vi "Begin.vi"(8 "error in":errorcluster) -> (0 "error out":errorcluster)   [LabVIEW 2020]
doc: "Called before other user functions, this VI is expected to open initial I/O refnums, load in file data, and do all program initialization. Notice that the <B>error out</B> terminal is simply used for data flow. Wiring it to other structures or subVIs ensures that this VI runs first."
uses:
  <vilib>/Rock Robotics/WPI/DriverStation/WPI_DriverStationRobotMode2.ctl
  <vilib>/Rock Robotics/WPI/Joystick/WPI_JoystickDeviceEnum.ctl
  <vilib>/Rock Robotics/WPI/RobotDrive/WPI_RobotDriveDevRef.ctl
  <vilib>/Rock Robotics/WPI/MotorControl/WPI_MotorControlDeviceRef.ctl
  <vilib>/Rock Robotics/WPI/MotorControl/WPI_MotorControlType.ctl
  <vilib>/Rock Robotics/SystemInterfaces/DIO/FPGA_DIOPWMChannel.ctl
  <vilib>/Rock Robotics/WPI/PWM/WPI_PWMDeadband.ctl
  <vilib>/Rock Robotics/SystemInterfaces/DIO/FPGA_DIOChannel.ctl
  <vilib>/Rock Robotics/WPI/SafetyOutput/WPI_SafetyOutputConfigMenu.ctl
  <vilib>/Rock Robotics/WPI/Solenoid/WPI_SolenoidChannel.ctl
  <vilib>/Rock Robotics/WPI/ThirdParty/REV Robotics/REVLib/Typedef/Spark MAX Idle Mode.ctl
  <vilib>/Rock Robotics/WPI/ThirdParty/REV Robotics/REVLib/Typedef/Spark MAX Motor Type.ctl
  Robot Global Data.vi
  <vilib>/Rock Robotics/Network Tables/NT Write String Array.vi
  <vilib>/Rock Robotics/WPI/Utilities/WPI_GetSetVariantRefNum.vi
  <vilib>/Rock Robotics/WPI/Solenoid/WPI_SolenoidOpenSingle.vi
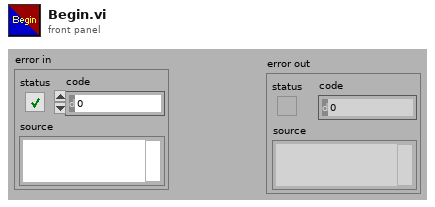
[diagram p1: front panel]
types:
  T1 = typedef "WPI_SafetyOutputConfigMenu.ctl" = enum16{"Enable", "Disable"}
  T2 = typedef "WPI_SolenoidChannel.ctl" = enum8{"Solenoid 0", "Solenoid 1", "Solenoid 2", "Solenoid 3", "Solenoid 4", "Solenoid 5", "Solenoid 6", "Solenoid 7", "Solenoid 8", "Solenoid 9", "Solenoid 10", "Solenoid 11", "Solenoid 12", "Solenoid 13", "Solenoid 14", "Solenoid 15", "Invalid"}
  T3 = typedef "WPI_JoystickDeviceEnum.ctl" = enum16{"USB 0", "USB 1", "USB 2", "USB 3", "USB 4", "USB 5"}
  T4 = typedef "WPI_RobotDriveDevRef.ctl" = cluster{"DevStatus":errorcluster, "Motors[]":T5[], "Square Inputs":bool, "Max Output":dbl}
  T5 = typedef "WPI_MotorControlDeviceRef.ctl" = cluster{"DeviceStatus":errorcluster, "Type":T6, "PWM":cluster{"PWM Channel":T7, "DeadBand":T8}, "CAN":cluster{"Device Number":u8, "SetOutput VI Ref":variant, "GetOutput VI Ref":variant, "Enable VI Ref":variant, "Disable VI Ref":variant, "Data":variant}, "Invert":bool, "DIO PWM":cluster{"PWM \"Enable\" Channel":T7, "DIOChannel":T9, "PWM Rate":dbl}}
  T6 = typedef "WPI_MotorControlType.ctl" = enum16{"PWM", "CAN", "DIO PWM"}
  T7 = typedef "FPGA_DIOPWMChannel.ctl" = enum8{"PWM 0", "PWM 1", "PWM 2", "PWM 3", "PWM 4", "PWM 5", "PWM 6", "PWM 7", "PWM 8", "PWM 9", "PWM MXP 0", "PWM MXP 1", "PWM MXP 2", "PWM MXP 3", "PWM MXP 4", "PWM MXP 5", "PWM MXP 6", "PWM MXP 7", "PWM MXP 8", "PWM MXP 9", "Invalid"}
  T8 = typedef "WPI_PWMDeadband.ctl" = cluster{"Name":string, "maxPositivePwm":i32, "minPositivePwm":i32, "centerPwm":i32, "maxNegativePwm":i32, "minNegativePwm":i32, "angularRange":u16}
  T9 = typedef "FPGA_DIOChannel.ctl" = enum8{"DIO 0", "DIO 1", "DIO 2", "DIO 3", "DIO 4", "DIO 5", "DIO 6", "DIO 7", "DIO 8", "DIO 9", "DIO MXP 0", "DIO MXP 1", "DIO MXP 2", "DIO MXP 3", "DIO MXP 4", "DIO MXP 5", "DIO MXP 6", "DIO MXP 7", "DIO MXP 8", "DIO MXP 9", "DIO MXP 10", "DIO MXP 11", "DIO MXP 12", "DIO MXP 13", "DIO MXP 14", "DIO MXP 15", "SPI Port CS1", "SPI Port CS2", "SPI Port CS3", "SPI Port MISO", "SPI Port MOSI", "Invalid"}
  T10 = typedef "WPI_DriverStationRobotMode2.ctl" = enum16{"Autonomous Disabled", "Autonomous Enabled", "Teleop Disabled", "Teleop Enabled", "Disconnected", "Finish", "Test Disabled", "Test Enabled", "Emergency Stopped"}
  T11 = typedef "WPI_SolenoidDevRef.ctl" = cluster{"DevStatus":errorcluster, "Pneumatics Control Module":u8, "Forward Solenoid Channel":T2, "Reverse Solenoid Channel":T2}
  T12 = typedef "WPI_CompressorDevRef.ctl" = cluster{"DevStatus":errorcluster, "Pneumatics Control Module":u8}
  T13 = typedef "WPI_JoystickDevRef.ctl" = cluster{"Device":T3}
  T14 = typedef "Spark MAX Motor Type.ctl" = enum16{"Brushed", "Brushless"}
  T15 = typedef "Spark MAX Idle Mode.ctl" = enum16{"Coast", "Brake"}
  T16 = cluster{"Motors[][0]":T5, "Motors[][1]":T5, "Motors[][2]":T5, "Motors[][3]":T5, "Motors[][4]":T5, "Motors[][5]":T5, "Motors[][6]":T5, "Motors[][7]":T5, "Motors[][8]":T5}
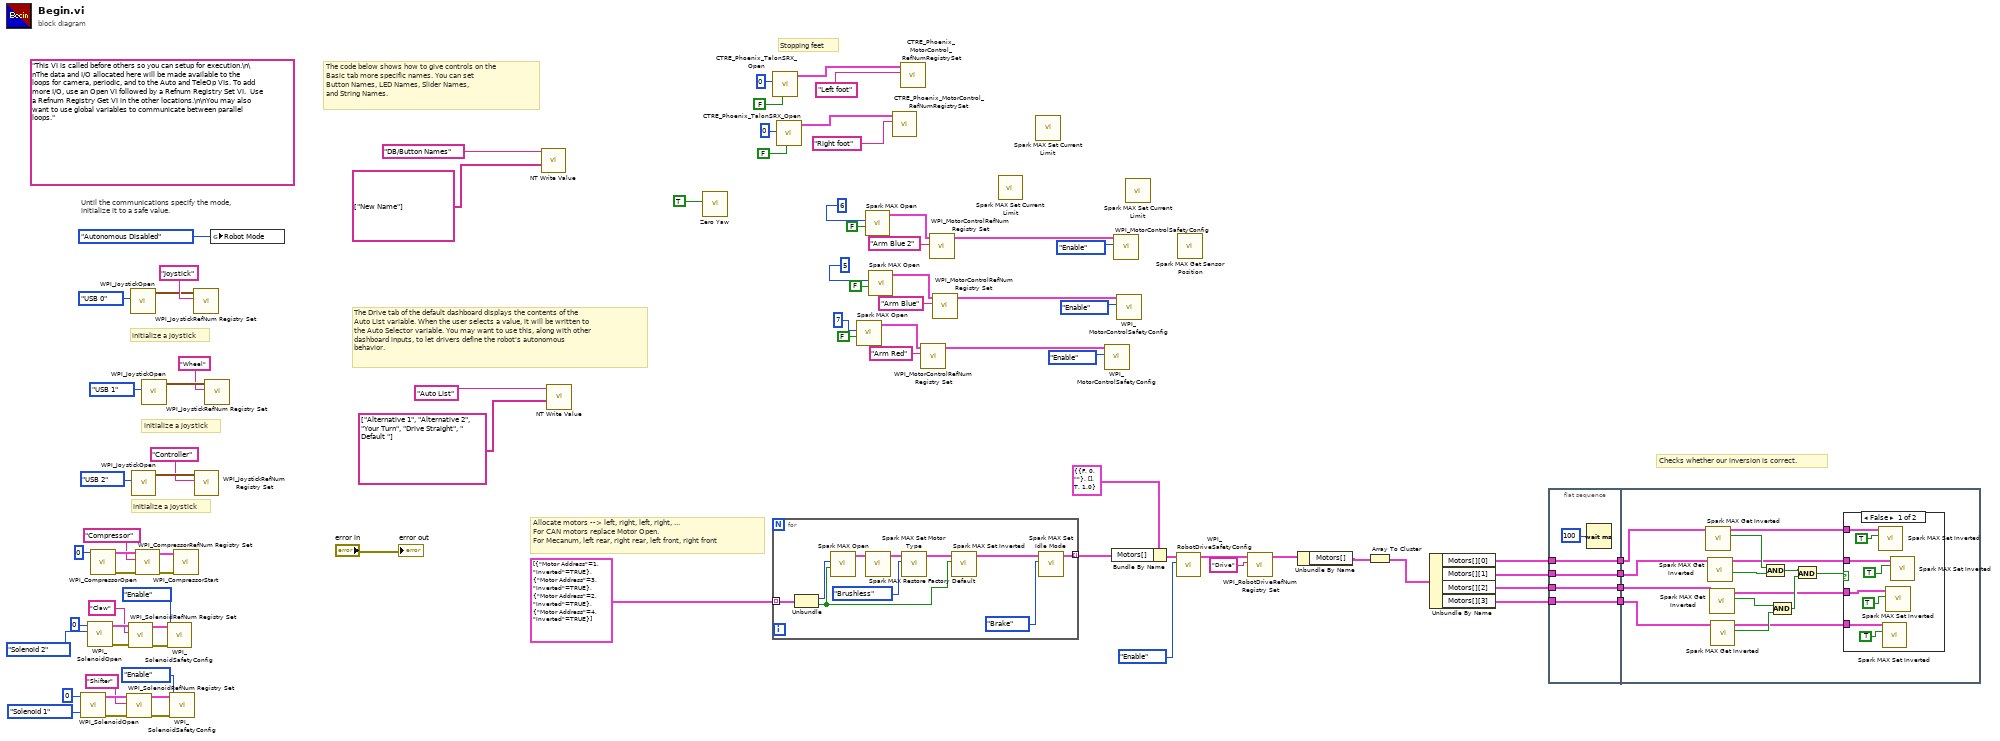
[diagram p0: block diagram]
diagram:
  (unwired) "This VI is called before others so you can setup for execution.\n\nThe data and I/O allocated here will be made available to the loops for camera, periodic, and to the Auto and TeleOp VIs. To add more I/O, use an Open VI followed by a Refnum Registry Set VI.  Use a Refnum Registry Get VI in the other locations.\n\nYou may also want to use global variables to communicate between parallel loops."
  # "Stopping feet"
  # "Checks whether our inversion is correct."
  # "initialize a joystick"
  # "initialize a joystick"
  # "Allocate motors --> left, right, left, right, ... \nFor CAN motors replace Motor Open.\nFor Mecanum, left rear, right rear, left front, right front"
  # "The Drive tab of the default dashboard displays the contents of the\nAuto List variable. When the user selects a value, it will be written to\nthe Auto Selector variable. You may want to use this, along with other\ndashboard inputs, to let drivers define the robot's autonomous\nbehavior."
  # "The code below shows how to give controls on the\nBasic tab more specific names. You can set\nButton Names, LED Names, Slider Names,\nand String Names."
  # "initialize a joystick"
  # "Until the communications specify the mode,\ninitialize it to a safe value."
  n1 = call-poly <vilib>:"WPI_SolenoidOpen.vi"("Solenoid Channel"=WPI_SolenoidChannel."Solenoid 1", "Pneumatics Device (def)"=u8 0) -> ("error out"=w39:errorcluster, "SolenoidDevRef"=w38:T11)  [unwired: 8 in]
  n2 = call-poly <vilib>:"WPI_SolenoidOpen.vi"("Solenoid Channel"=WPI_SolenoidChannel."Solenoid 2", "Pneumatics Device (def)"=u8 0) -> ("error out"=w41:errorcluster, "SolenoidDevRef"=w40:T11)  [unwired: 8 in]
  n3 = call <vilib>:"WPI_CompressorOpen.vi"("Pneumatics device (def)"=u8 0) -> ("CompressorDevRef"=w46:T12, "error out"=w47:errorcluster)  [unwired: 13 in]
  n4 = call <vilib>:"WPI_SolenoidRefNum Registry Set.vi"("error in (no error)"=w39, "refnum name"="Shifter", "SolenoidDevRef"=w38) -> ("error out"=w30:errorcluster, "SolenoidDevRef"=w29:T11)  [unwired: 7 in]
  n5 = call <vilib>:"WPI_SolenoidRefNum Registry Set.vi"("error in (no error)"=w41, "refnum name"="Claw", "SolenoidDevRef"=w40) -> ("error out"=w33:errorcluster, "SolenoidDevRef"=w32:T11)  [unwired: 7 in]
  n6 = call <vilib>:"WPI_JoystickOpen.vi"("JoystickDevice"=WPI_JoystickDeviceEnum."USB 0") -> ("JoystickDevRef"=w80:T13)  [unwired: 10 in]
  n7 = call <vilib>:"WPI_JoystickOpen.vi"("JoystickDevice"=WPI_JoystickDeviceEnum."USB 2") -> ("JoystickDevRef"=w63:T13)  [unwired: 10 in]
  n8 = call <vilib>:"WPI_CompressorRefNum Registry Set.vi"("error in (no error)"=w47, "refnum name"="Compressor", "CompressorDevRef"=w46) -> ("error out"=w43:errorcluster, "CompressorDevRef"=w42:T12)  [unwired: 7 in]
  n9 = call <vilib>:"WPI_JoystickOpen.vi"("JoystickDevice"=WPI_JoystickDeviceEnum."USB 1") -> ("JoystickDevRef"=w66:T13)  [unwired: 10 in]
  n10 = call <vilib>:"WPI_SolenoidSafetyConfig.vi"("error in (no error)"=w33, "mode"=WPI_SafetyOutputConfigMenu."Enable", "SolenoidDevRef"=w32) -> ()  [unwired: 7 in, 2 out]
  n11 = call <vilib>:"WPI_SolenoidSafetyConfig.vi"("error in (no error)"=w30, "mode"=WPI_SafetyOutputConfigMenu."Enable", "SolenoidDevRef"=w29) -> ()  [unwired: 7 in, 2 out]
  n12 = call <vilib>:"WPI_CompressorStart.vi"("error in (no error)"=w43, "CompressorDevRef"=w42) -> ()  [unwired: 8 in, 2 out]
  n13 = call <vilib>:"WPI_JoystickRefNum Registry Set.vi"("refnum name"="Joystick", "JoystickDevRef"=w80) -> ()  [unwired: 8 in, 2 out]
  n14 = call <vilib>:"WPI_JoystickRefNum Registry Set.vi"("refnum name"="Controller", "JoystickDevRef"=w63) -> ()  [unwired: 8 in, 2 out]
  n15 = call <vilib>:"WPI_JoystickRefNum Registry Set.vi"("refnum name"="Wheel", "JoystickDevRef"=w66) -> ()  [unwired: 8 in, 2 out]
  n16 = global write "Robot Global Data.vi" "Robot Mode"(WPI_DriverStationRobotMode2."Autonomous Disabled" ("Robot Mode")) -> ()
  n17 = call-poly <vilib>:"NT Write Value.vi"("value"=string[] ["New Name"], "name"="DB/Button Names" ("Name")) -> ()  [unwired: 9 in, 1 out]
  n18 = call-poly <vilib>:"NT Write Value.vi"("value"=string[] ["Alternative 1", "Alternative 2", "Your Turn", "Drive Straight", " Default "] ("String Array"), "name"="Auto List" ("Name")) -> ()  [unwired: 9 in, 1 out]
  n19 = call <vilib>:"Zero Yaw.vi"("Zero"=TRUE) -> ()  [unwired: 11 in]
  n20 = call <vilib>:"CTRE_Phoenix_TalonSRX_Open.vi"("Invert"=FALSE, "Device Number"=u8 0) -> ("PhoenixMotorControlDevRef"=w8:T5)  [unwired: 8 in, 1 out]
  n21 = for {
    tunnel: cluster{"Motor Address":i32, "Inverted":bool}[] [{"Motor Address"=1, "Inverted"=TRUE}, {"Motor Address"=3, "Inverted"=TRUE}, {"Motor Address"=2, "Inverted"=TRUE}, {"Motor Address"=4, "Inverted"=TRUE}] ("Array") -> [w92] mode=indexing
    tunnel: [w89] -> w48 mode=indexing
    n22 = Unbundle(w92) -> ("Motor Address"=w91:i32, "Inverted"=w84:bool)
    n23 = call <vilib>:"Spark MAX Open.vi"("Invert"=w84, "Device Number"=w91) -> ("MotorControlDeviceRef"=w88:T5)  [unwired: 8 in, 1 out]
    n24 = call <vilib>:"Spark MAX Restore Factory Default.vi"("MotorControlDeviceRef"=w88) -> ("MotorControlDeviceRef"=w87:T5)  [unwired: 9 in, 1 out]
    n25 = call <vilib>:"Spark MAX Set Motor Type.vi"("Motor Type"=Spark_MAX_Motor_Type."Brushless", "MotorControlDevRef"=w87) -> ("MotorControlDeviceRef"=w86:T5)  [unwired: 8 in, 1 out]
    n26 = call <vilib>:"Spark MAX Set Inverted.vi"("Inverted (F)"=w84, "MotorControlDeviceRef in"=w86) -> ("MotorControlDeviceRef out"=w85:T5)  [unwired: 8 in, 1 out]
    n27 = call <vilib>:"Spark MAX Set Idle Mode.vi"("Idle Mode"=Spark_MAX_Idle_Mode."Brake", "MotorControlDeviceRef in"=w85) -> ("MotorControlDeviceRef out"=w89:T5)  [unwired: 8 in, 1 out]
  }
  n28 = call <vilib>:"CTRE_Phoenix_TalonSRX_Open.vi"("Invert"=FALSE, "Device Number"=u8 0) -> ("PhoenixMotorControlDevRef"=w5:T5)  [unwired: 8 in, 1 out]
  n29 = call <vilib>:"Spark MAX Open.vi"("Invert"=FALSE, "Device Number"=u8 7) -> ("MotorControlDeviceRef"=w60:T5)  [unwired: 8 in, 1 out]
  n30 = call <vilib>:"Spark MAX Open.vi"("Invert"=FALSE, "Device Number"=u8 6) -> ("MotorControlDeviceRef"=w23:T5)  [unwired: 8 in, 1 out]
  n31 = call <vilib>:"Spark MAX Open.vi"("Invert"=FALSE, "Device Number"=u8 5) -> ("MotorControlDeviceRef"=w53:T5)  [unwired: 8 in, 1 out]
  n32 = call <vilib>:"CTRE_Phoenix_MotorControl_RefNumRegistrySet.vi"("refnum name"="Right foot", "PhoenixMotorControlDevRef"=w5) -> ()  [unwired: 8 in, 2 out]
  n33 = call <vilib>:"CTRE_Phoenix_MotorControl_RefNumRegistrySet.vi"("refnum name"="Left foot", "PhoenixMotorControlDevRef"=w8) -> ()  [unwired: 8 in, 2 out]
  n34 = call <vilib>:"WPI_MotorControlRefNum Registry Set.vi"("refnum name"="Arm Red", "MotorControlDevRef"=w60) -> ("MotorControlDevRef"=w57:T5)  [unwired: 8 in, 1 out]
  n35 = call <vilib>:"WPI_MotorControlRefNum Registry Set.vi"("refnum name"="Arm Blue 2", "MotorControlDevRef"=w23) -> ("MotorControlDevRef"=w20:T5)  [unwired: 8 in, 1 out]
  n36 = call <vilib>:"WPI_MotorControlRefNum Registry Set.vi"("refnum name"="Arm Blue", "MotorControlDevRef"=w53) -> ("MotorControlDevRef"=w56:T5)  [unwired: 8 in, 1 out]
  n37 = call <vilib>:"Spark MAX Set Current Limit.vi"() -> ()  [unwired: 10 in, 2 out]
  n38 = call <vilib>:"Spark MAX Set Current Limit.vi"() -> ()  [unwired: 10 in, 2 out]
  n39 = call <vilib>:"WPI_MotorControlSafetyConfig.vi"("mode"=WPI_SafetyOutputConfigMenu."Enable", "MotorControlDevRef"=w57) -> ()  [unwired: 8 in, 2 out]
  n40 = Bundle By Name(cluster=T4 {"DevStatus"={"status"=FALSE, "code"=0, "source"=""}, "Motors[]"=[], "Square Inputs"=TRUE, "Max Output"=1.0} ("RobotDriveDevRef"), "Motors[]"=w48) -> (w72:T4)
  n41 = call <vilib>:"WPI_MotorControlSafetyConfig.vi"("mode"=WPI_SafetyOutputConfigMenu."Enable", "MotorControlDevRef"=w20) -> ()  [unwired: 8 in, 2 out]
  n42 = call <vilib>:"WPI_MotorControlSafetyConfig.vi"("mode"=WPI_SafetyOutputConfigMenu."Enable", "MotorControlDevRef"=w56) -> ()  [unwired: 8 in, 2 out]
  n43 = call <vilib>:"Spark MAX Set Current Limit.vi"() -> ()  [unwired: 10 in, 2 out]
  n44 = call <vilib>:"WPI_RobotDriveSafetyConfig.vi"("mode"=WPI_SafetyOutputConfigMenu."Enable", "RobotDriveDevRef"=w72) -> ("RobotDriveDevRef"=w69:T4)  [unwired: 2 in, 7 out]
  n45 = call <vilib>:"Spark MAX Get Sensor Position.vi"() -> ()  [unwired: 8 in, 4 out]
  n46 = call <vilib>:"WPI_RobotDriveRefNum Registry Set.vi"("refnum name"="Drive", "RobotDriveDevRef"=w69) -> ("RobotDriveDevRef"=w17:T4)  [unwired: 8 in, 1 out]
  n47 = Unbundle By Name(w17) -> ("Motors[]"=w19:T5[])
  n48 = Array To Cluster(array=w19) -> (cluster=w18:T16)
  n49 = Unbundle By Name(w18) -> ("Motors[][0]"=w15:T5, "Motors[][1]"=w13:T5, "Motors[][2]"=w11:T5, "Motors[][3]"=w9:T5)
  n50 = flat-sequence {
    tunnel: [w96] -> w16
    tunnel: w15 -> [w96]
    tunnel: [w95] -> w14
    tunnel: w13 -> [w95]
    tunnel: [w94] -> w12
    tunnel: w11 -> [w94]
    tunnel: [w93] -> w10
    tunnel: w9 -> [w93]
    tunnel: w16 -> [w101]
    tunnel: w14 -> [w100]
    tunnel: w12 -> [w99]
    tunnel: w10 -> [w98]
    frame #0 {
      n51 = Wait (ms)(milliseconds to wait=u32 100) -> ()  [unwired: 1 out]
    }
    frame #1 {
      n52 = call <vilib>:"Spark MAX Get Inverted.vi"("MotorControlDeviceRef in"=w101) -> ("Inverted"=w112:bool, "MotorControlDeviceRef out"=w105:T5)  [unwired: 8 in, 1 out]
      n53 = call <vilib>:"Spark MAX Get Inverted.vi"("MotorControlDeviceRef in"=w100) -> ("Inverted"=w111:bool, "MotorControlDeviceRef out"=w104:T5)  [unwired: 8 in, 1 out]
      n54 = call <vilib>:"Spark MAX Get Inverted.vi"("MotorControlDeviceRef in"=w99) -> ("Inverted"=w110:bool, "MotorControlDeviceRef out"=w103:T5)  [unwired: 8 in, 1 out]
      n55 = call <vilib>:"Spark MAX Get Inverted.vi"("MotorControlDeviceRef in"=w98) -> ("Inverted"=w109:bool, "MotorControlDeviceRef out"=w102:T5)  [unwired: 8 in, 1 out]
      n56 = And(x=w112, y=w111) -> (x .and. y?=w107:bool)
      n57 = And(x=w110, y=w109) -> (x .and. y?=w108:bool)
      n58 = And(x=w107, y=w108) -> (x .and. y?=w106:bool)
      n59 = case shown="False" w106 {
        tunnel: w105 -> [w120 _]
        tunnel: w104 -> [w119 _]
        tunnel: w103 -> [w118 _]
        tunnel: w102 -> [w117 _]
        frame False {
          n60 = call <vilib>:"Spark MAX Set Inverted.vi"("Inverted (F)"=TRUE, "MotorControlDeviceRef in"=w120) -> ()  [unwired: 8 in, 2 out]
          n61 = call <vilib>:"Spark MAX Set Inverted.vi"("Inverted (F)"=TRUE, "MotorControlDeviceRef in"=w117) -> ()  [unwired: 8 in, 2 out]
          n62 = call <vilib>:"Spark MAX Set Inverted.vi"("Inverted (F)"=TRUE, "MotorControlDeviceRef in"=w118) -> ()  [unwired: 8 in, 2 out]
          n63 = call <vilib>:"Spark MAX Set Inverted.vi"("Inverted (F)"=TRUE, "MotorControlDeviceRef in"=w119) -> ()  [unwired: 8 in, 2 out]
        }
        frame True {
        }
      }
    }
  }
  "error out" <- "error in"
